vi "Abort Test.vi"(8 "error in (no error)":errorcluster, 11 "TestStand Adapter in":refnum<class "TestStand Adapter.lvclass">) -> (0 "error out":errorcluster, 3 "TestStand Adapter out":refnum<class "TestStand Adapter.lvclass">)   [LabVIEW 2026, in "TestStand Adapter.lvclass"]
uses:
  TestStand Adapter.lvclass
  TestStand Adapter.lvclass/TestStand Adapter.ctl
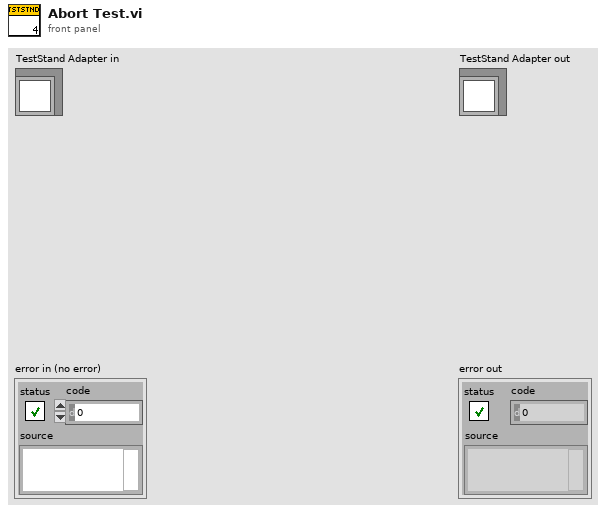
[diagram p1: front panel]
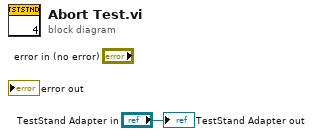
[diagram p0: block diagram]
diagram:
  "TestStand Adapter out" <- "TestStand Adapter in"
